vi "in_Lagrange scaled Y values.vi"(10 "X[0..N]":dbl[](array[numeric]) format="%_6g", 11 "Y[0..N]":dbl[](array[numeric]) format="%_6g") -> (3 "scaled Y":dbl[](array[numeric]) format="%_6g")   [LabVIEW 2011, in "NI_Gmath.lvlib"]
uses:
  NI_Gmath.lvlib
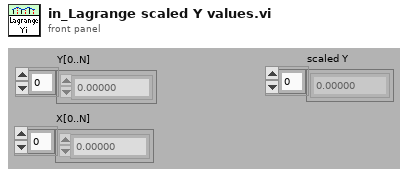
[diagram p1: front panel]
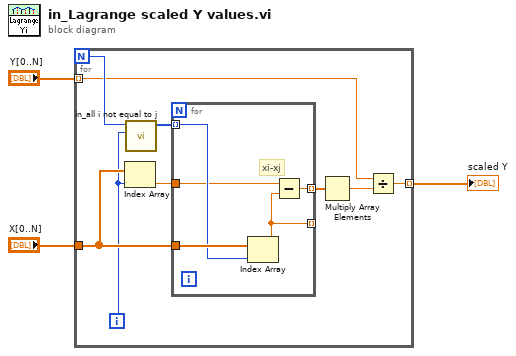
[diagram p0: block diagram]
diagram:
  n1 = for {
    N -> [w12]
    tunnel: "Y[0..N]" -> [w8] mode=indexing
    tunnel: "X[0..N]" -> [w7]
    tunnel: [w5] -> w1 mode=indexing
    i -> [w4]
    n2 = Index Array(array=w7, index=w4) -> (element=w6:dbl)
    n3 = call "in_all i not equal to j.vi"("index"=w4, "N"=w12) -> ("index values"=w11:i32[])  [unwired: 9 in]
    n4 = for {
      tunnel: w11 -> [w16] mode=indexing
      tunnel: w7 -> [w17]
      tunnel: w6 -> [w15]
      tunnel: [w14] -> w10 mode=indexing
      tunnel: [w13] -> _ mode=indexing
      # "xi-xj"
      n5 = Index Array(array=w17, index=w16) -> (element=w13:dbl)
      n6 = Subtract(x=w15, y=w13) -> (x-y=w14:dbl)
    }
    n7 = Multiply Array Elements(1:w10) -> (0:w9:dbl)
    n8 = Divide(x=w8, y=w9) -> (x/y=w5:dbl)
  }
  "scaled Y" <- w1
